vi "GUI_AndorCamera.vi"() -> ()   [LabVIEW 2020]
uses:
  Shared/GUI_Template/GUI_master/tcp_new_data_event.ctl
  Shared/GUI_Template/GUI_master/tcp new data cluster.ctl
  <vilib>/vision/NI_Vision_Development_Module.lvlib
panel:
  in  "multiplier":dbl=1.0 format="%.2f"
  in  "Refresh Button":bool
  in  "Select device":string(combo)="PL1-PresCtl"
  out "Waveform Chart":sgl(graph)
  in  "trigger::1":enum16{"Internal", "External"}(ring) caption="trigger"
  in  "pulsewidth::1":dbl caption="Pulse Width (ns)" min=0.0 max=1000000000.0
  in  "gain::1":dbl caption="gain" min=0.0 max=4095.0
  in  "temperature::1":dbl caption="Temperature (C)" min=-40.0 max=20.0
  in  "acqready::1":enum16{"yes", "no"}(ring)
  in  "stop":bool
  in  "GUIdevice 1":string="P2-AndorCam"
  out "tcp data event":T1
  in  "Tab Control":enum32{"original", "Scaled", "As Graph"}(tab)
  out "image::1":T2(plugin-control) caption="Andor Camera"
  out "andorscaled":T2(plugin-control) caption="Andor Camera"
  out "Intensity Graph":u8[][](graph)
  # "To get chart to plot, select an roi on scaled image"
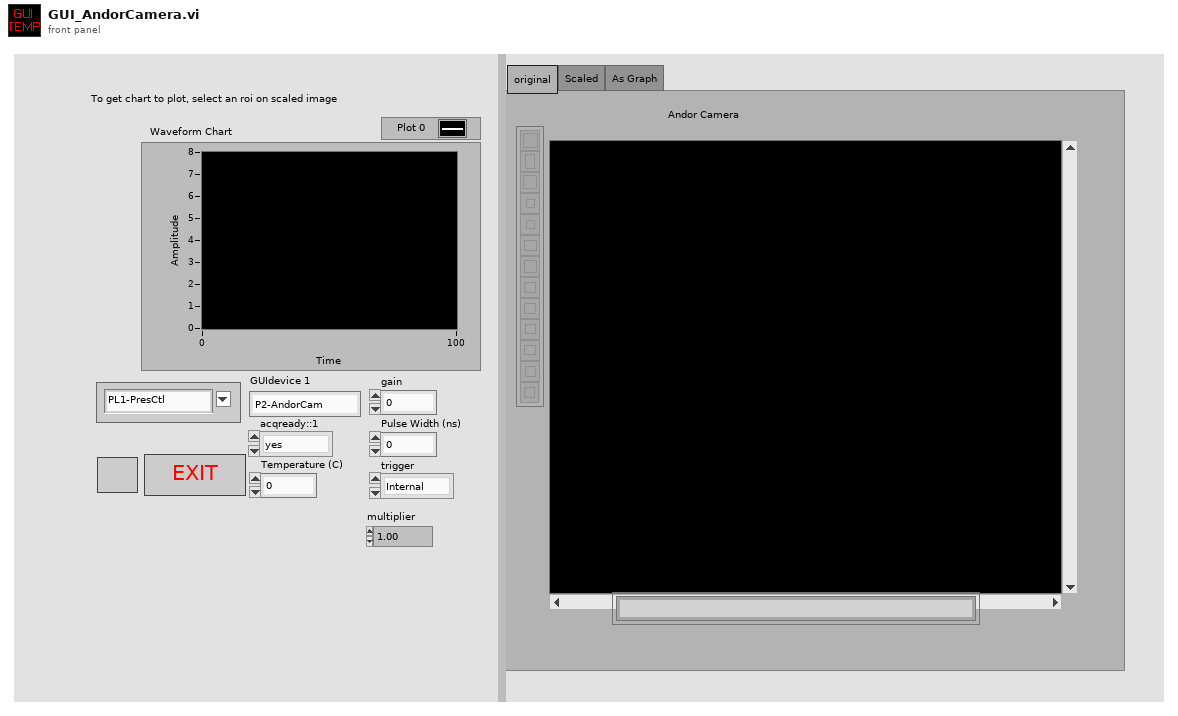
[diagram p1: front panel]
types:
  T1 = typedef "tcp_new_data_event.ctl" = refnum<user-event>
  T2 = typedef "IMAQ Image.ctl" = refnum<image>
  T3 = typedef "Image Type" = u32
  T4 = enum32{"invalid app kind", "Development System", "Run Time System", "Student Edition", "Embedded LabVIEW", "Evaluation", "Custom"}
  T5 = typedef "tcp new data cluster.ctl" = cluster{"EventEnum":enum16{"new data", "connection status update"}, "Device name":string}
  T6 = enum32{"Invalid", "Standard", "Closed", "Hidden", "Minimized", "Maximized"}
  T7 = cluster{"Core":cluster{"Current VI Reference":refnum<vi>, "Close Panel on Exit?":bool}, "SuperGUI":cluster{"STOP queue":refnum<queue>, "SuperGUI ref":refnum<vi>}}
  T8 = cluster{"STOP queue":refnum<queue>, "SuperGUI ref":refnum<vi>}
  T9 = cluster{"Current VI Reference":refnum<vi>, "Close Panel on Exit?":bool}
  T10 = cluster{"Global Rectangle":i32[], "Contours":cluster{"Contour Type":u32, "ROI Type":u32, "Points":i32[]}[]}
  T11 = cluster{"histogram":u32[], "Minimal Value":sgl, "Maximal Value":sgl, "Starting Value":sgl, "Interval Width":sgl, "Mean Value":sgl, "Standard  Variation":sgl, "Area (pixels)":i32}
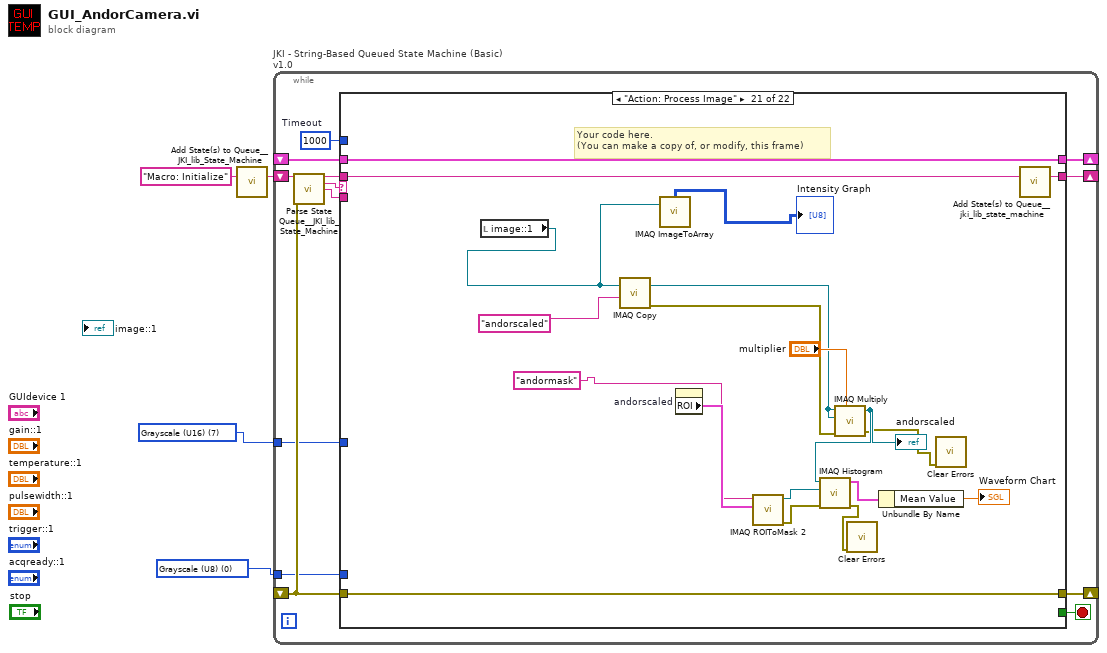
[diagram p0: block diagram]
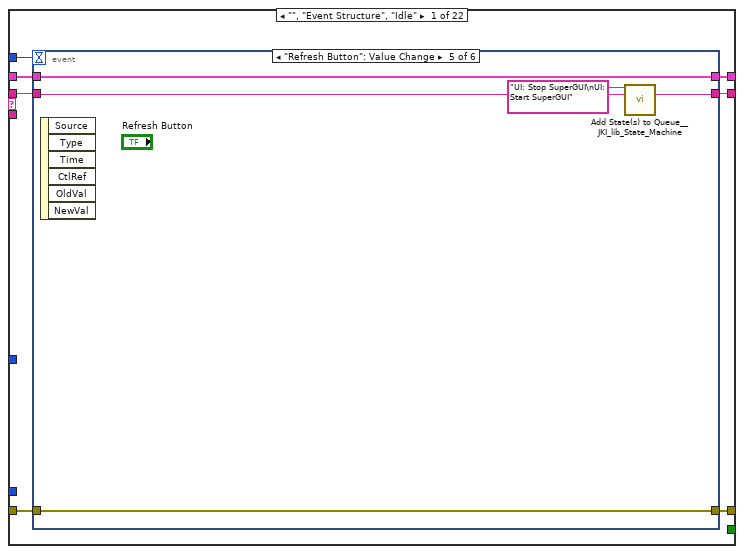
[diagram p2: hidden frame]
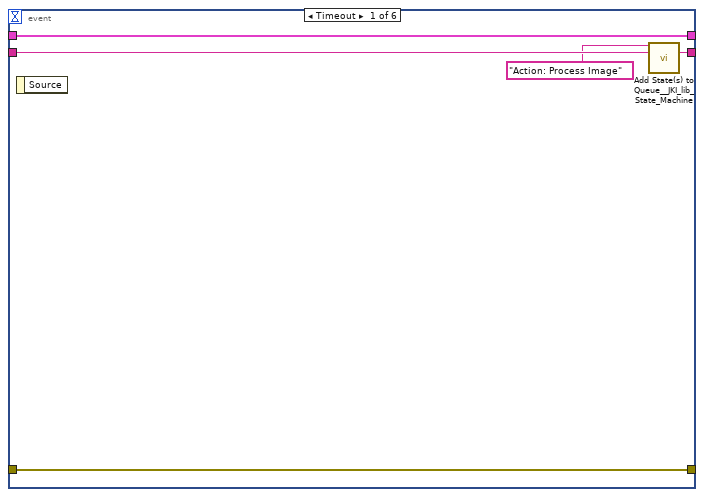
[diagram p3: hidden frame]
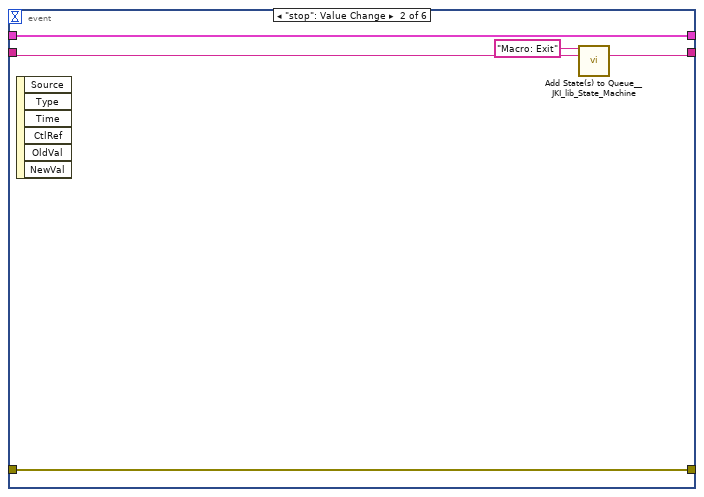
[diagram p4: hidden frame]
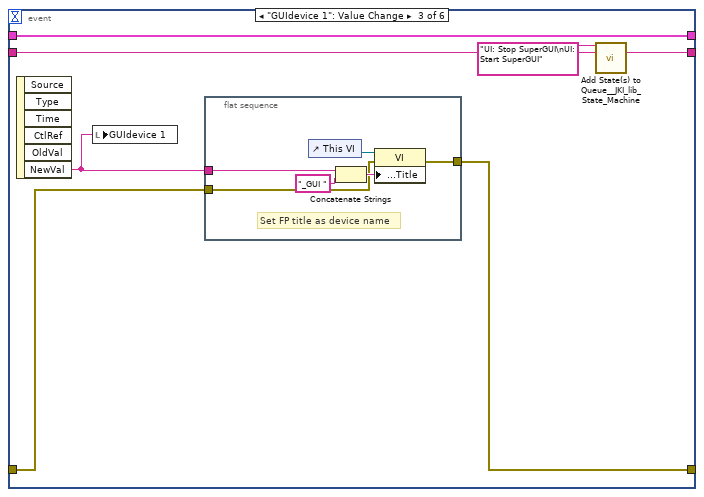
[diagram p5: hidden frame]
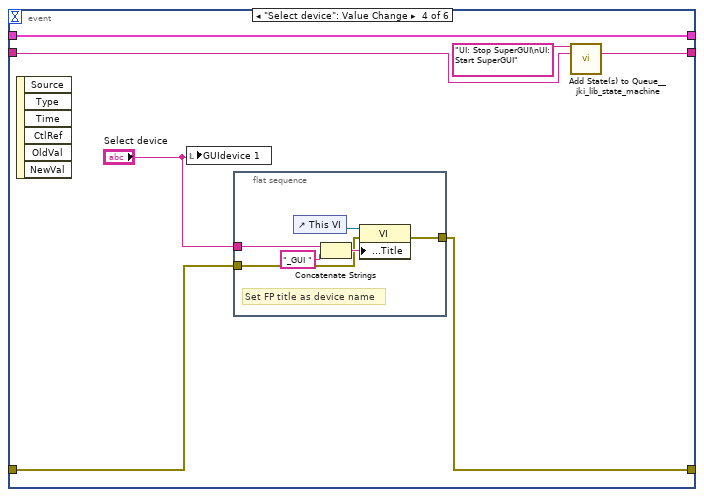
[diagram p6: hidden frame]
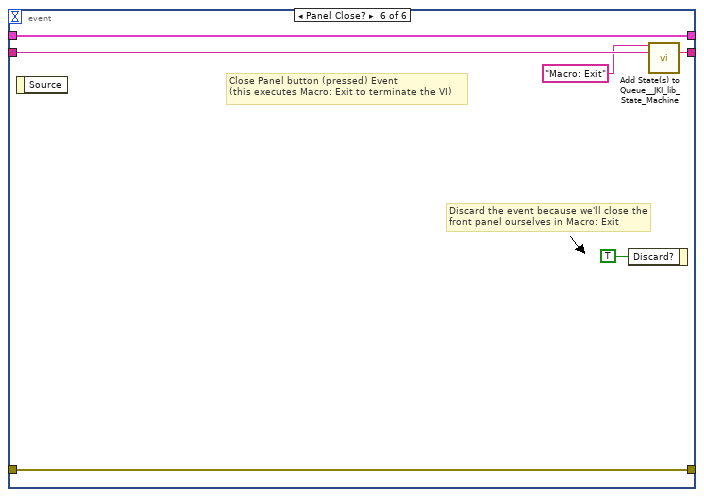
[diagram p7: hidden frame]
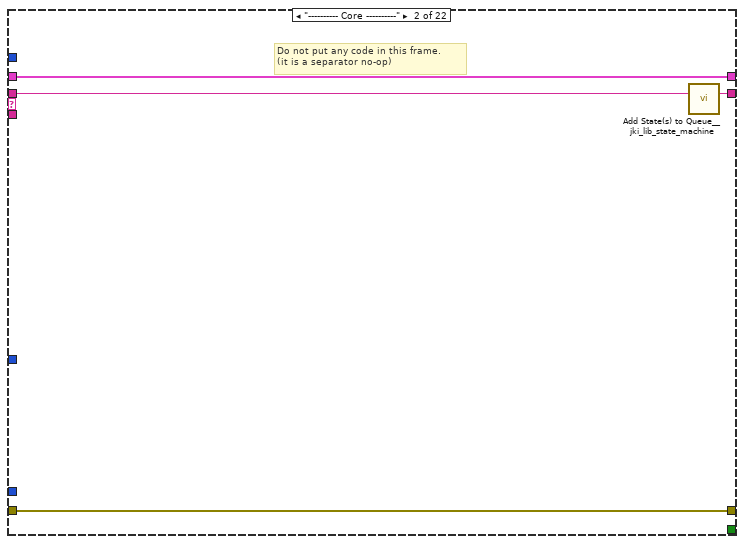
[diagram p8: hidden frame]
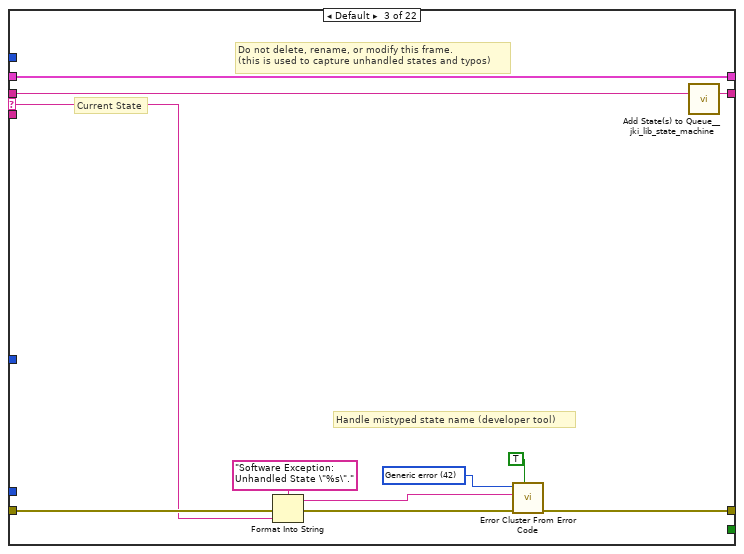
[diagram p9: hidden frame]
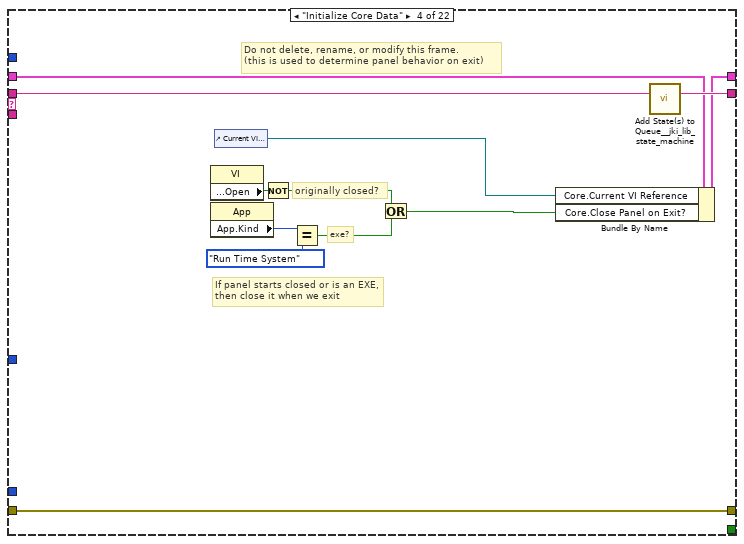
[diagram p10: hidden frame]
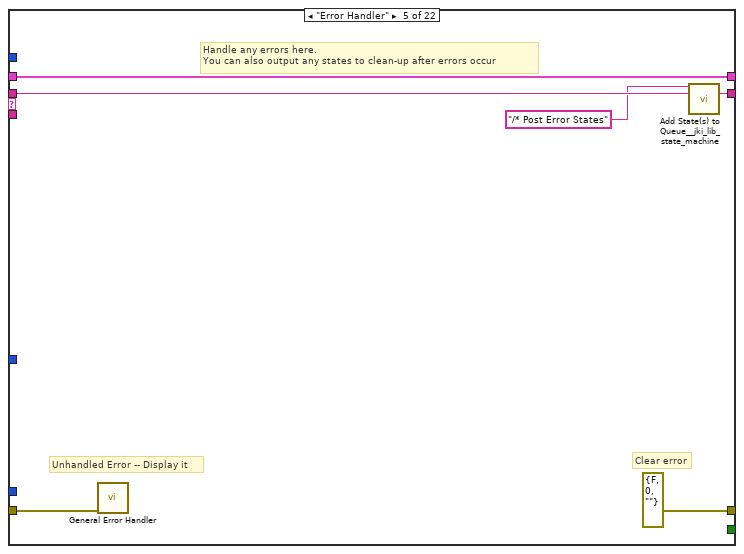
[diagram p11: hidden frame]
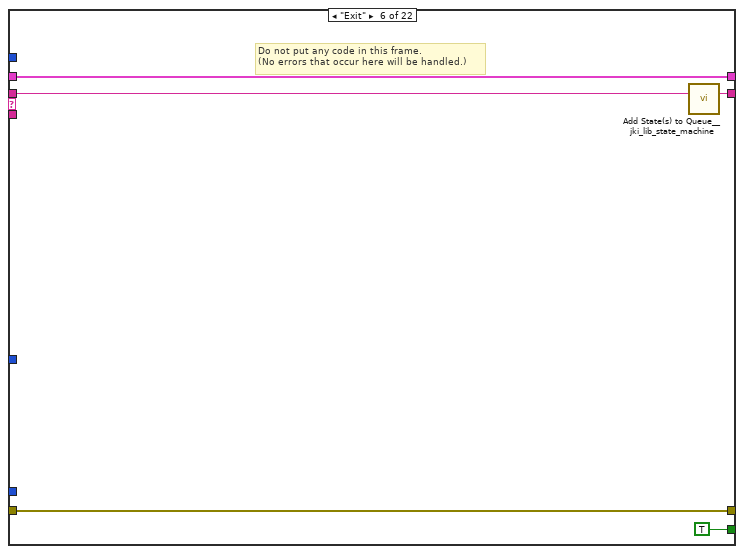
[diagram p12: hidden frame]
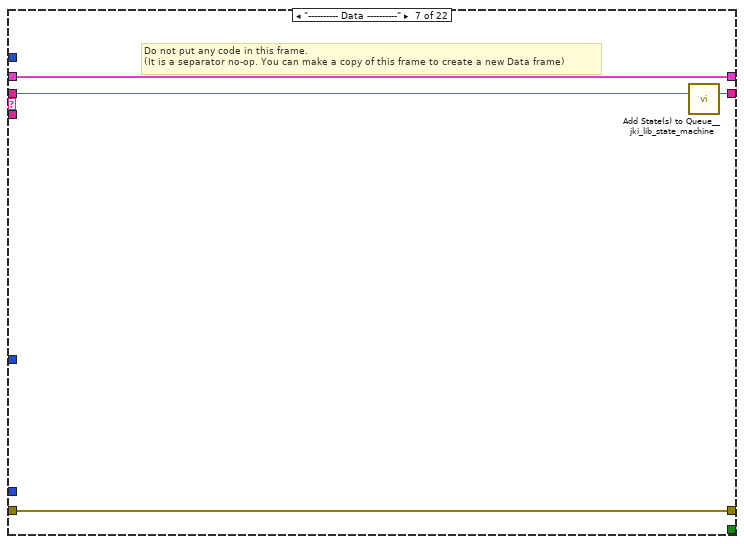
[diagram p13: hidden frame]
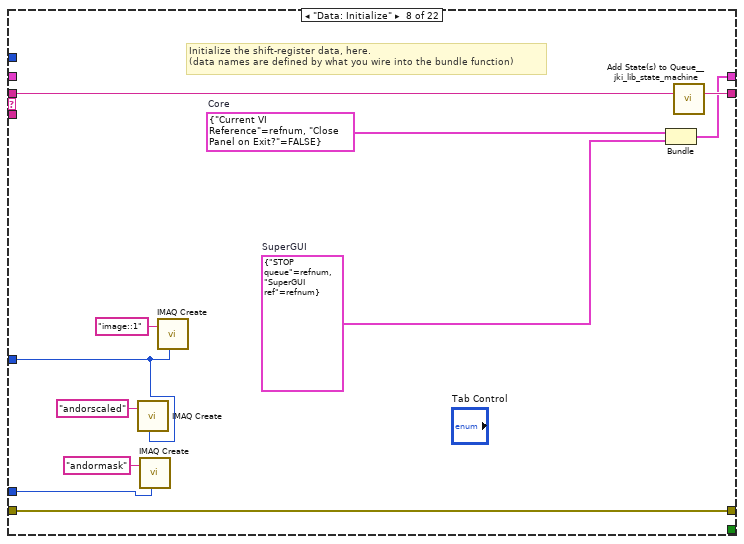
[diagram p14: hidden frame]
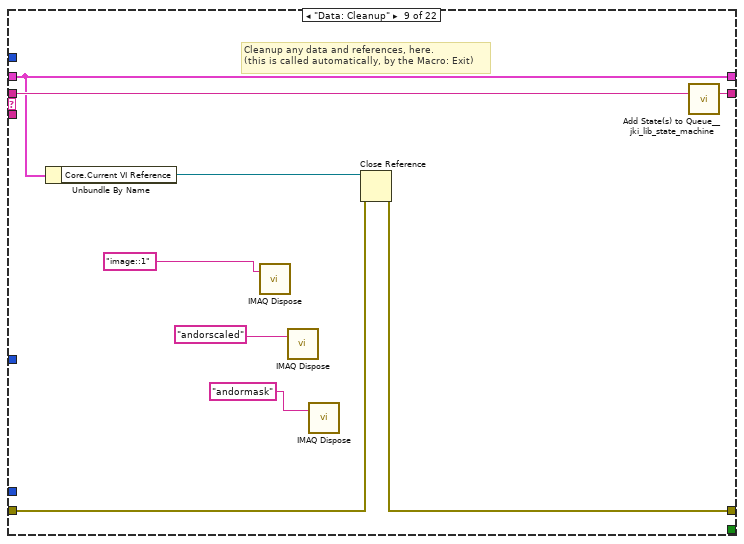
[diagram p15: hidden frame]
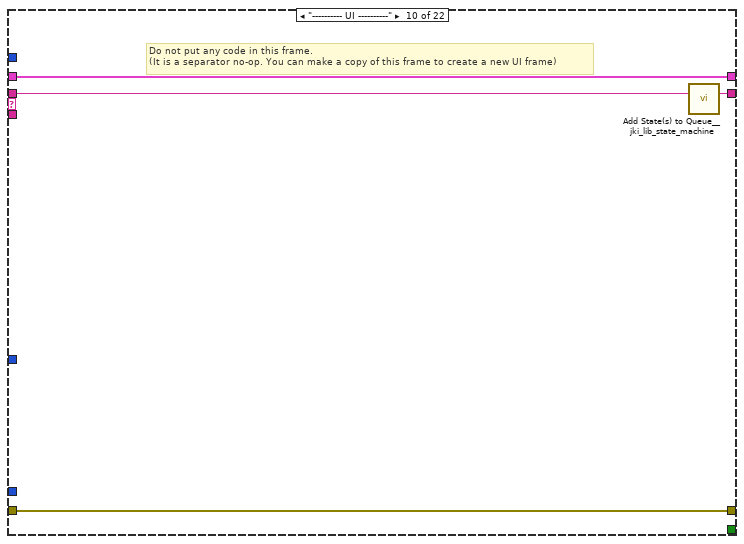
[diagram p16: hidden frame]
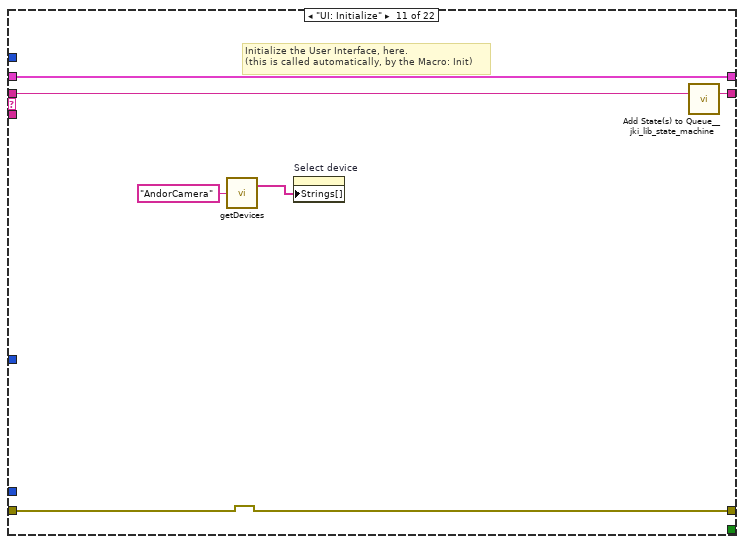
[diagram p17: hidden frame]
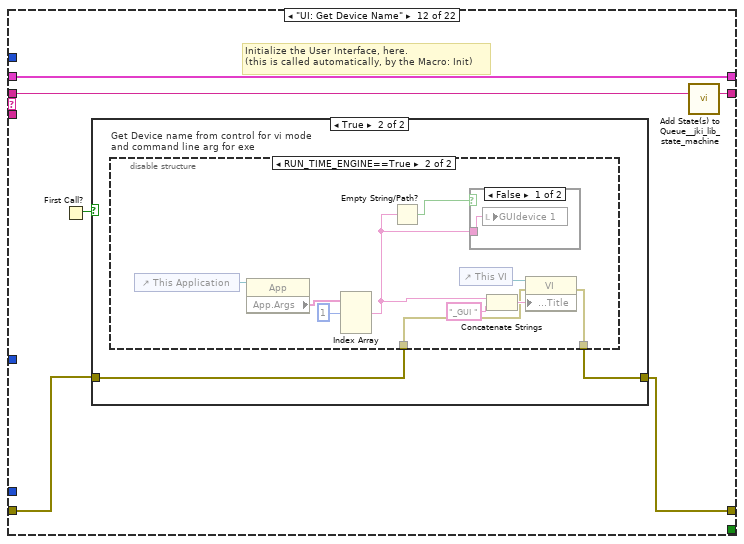
[diagram p18: hidden frame]
diagram:
  w1 = T3 0 items=["Grayscale (U8)", "Grayscale (I16)", "Grayscale (SGL)", "Complex (CSG)", "RGB (U32)", "HSL (U32)", "RGB (U64)", "Grayscale (U16)"] ("Image Type")
  w2 = T3 7 items=["Grayscale (U8)", "Grayscale (I16)", "Grayscale (SGL)", "Complex (CSG)", "RGB (U32)", "HSL (U32)", "RGB (U64)", "Grayscale (U16)"] ("Image Type")
  n1 = call <vilib>:"Add State(s) to Queue__JKI_lib_State_Machine.vi"("State(s) in (\"\")"="Macro: Initialize") -> ("States Out"=w4:string)  [unwired: 14 in]
  n2 = while "JKI - String-Based Queued State Machine (Basic) v1.0" {
    shift-right: [w10] -> _
    shift-left: _ -> [w9]
    shift-right: [w13] -> _
    shift-left: _ -> [w7]
    shift-right: [w12] -> _
    shift-left: w4 -> [w14]
    tunnel: w2 -> [w6]
    tunnel: w1 -> [w5]
    stop <- w11 stop-if-true
    w8 = 1000  # Timeout
    n3 = call <vilib>:"Parse State Queue__JKI_lib_State_Machine.vi"("State Queue"=w14, "Error In (no error)"=w7) -> ("Remaining States"=w16:string, "Current State"=w17:string, "Arguments"=w15:string)  [unwired: 11 in]
    n4 = case shown="\"Action: Process Image\"" w17 {
      selector: w17 -> [_ _ w76 _ _ _ _ _ _ _ _ _ _ _ _ _ _ _ _ _ _ _]
      tunnel: w16 -> [w24 w75 w80 w98 w104 w109 w113 w124 w133 w137 w143 w149 w184 w192 w198 w209 w235 w240 w250 w254 w273 w277]
      tunnel: w15 -> [_ _ _ _ _ _ _ _ _ _ _ _ _ _ w193 w203 _ _ _ _ _ _]
      tunnel: w9 -> [w22 w72 w78 w89 w101 w107 w110 _ w128 w134 w141 w147 w175 w187 w196 w205 w232 w237 w247 w251 w270 w274]
      tunnel: [w21 w73 w82 w95 errorcluster {"status"=FALSE, "code"=0, "source"=""} ("error out") w106 w111 w121 w129 w135 w138 w144 w168 w185 w194 w206 w233 w238 w248 w252 w271 w275] -> w13
      tunnel: w7 -> [w20 w73 w81 w95 w100 w106 w111 w121 w130 w135 w138 w145 w169 w186 w195 w207 w233 w238 w248 w252 w271 w275]
      tunnel: [w23 w74 w79 w97 w103 w108 w112 w123 w132 w136 w142 w148 w183 w191 w197 w208 w234 w239 w249 w253 w272 w276] -> w12
      tunnel: [_ _ _ _ _ TRUE _ _ _ _ _ _ _ _ _ _ _ _ _ _ _ _] -> w11
      tunnel: [w19 w72 w78 w96 w101 w107 w110 w122 w128 w134 w141 w147 w174 w187 w196 w205 w232 w237 w247 w251 w270 w274] -> w10
      tunnel: w8 -> [w18 _ _ _ _ _ _ _ _ _ _ _ _ _ _ _ _ _ _ _ _ _]
      tunnel: w6 -> [_ _ _ _ _ _ _ w115 _ _ _ _ _ _ _ _ _ _ _ _ _ _]
      tunnel: w5 -> [_ _ _ _ _ _ _ w114 _ _ _ _ _ _ _ _ _ _ _ _ _ _]
      frame "", "Event Structure", "Idle" {
        n5 = event shown="[4] \"Refresh Button\": Value Change" {
          selector: _ -> [_ _ _ _ _ _]
          dyn-events: _ -> [_ _ _ _ _ _]
          timeout: w18 -> [_ _ _ _ _ _]
          tunnel: w24 -> [w29 w32 w38 w49 w63 w71]
          tunnel: [w28 w31 w37 w48 w62 w70] -> w23
          tunnel: w22 -> [w26 w34 w41 w54 w65 w68]
          tunnel: [w27 w33 w39 w51 w64 w69] -> w21
          tunnel: w20 -> [w27 w33 w40 w52 w64 w69]
          tunnel: [w26 w34 w41 w54 w65 w68] -> w19
          event Timeout {
            n6 = event-data() -> ()  [unwired: 1 in, 1 out]
            n7 = call <vilib>:"Add State(s) to Queue__JKI_lib_State_Machine.vi"("State(s) in Front (\"\")"="Action: Process Image" ("State(s) in Front (\"\")"), "State(s) in (\"\")"=w29) -> ("States Out"=w28:string)  [unwired: 13 in]
          }
          event "stop": Value Change {
            n8 = event-data() -> ()  [unwired: 1 in, 6 out]
            n9 = call <vilib>:"Add State(s) to Queue__JKI_lib_State_Machine.vi"("State(s) in Front (\"\")"="Macro: Exit", "State(s) in (\"\")"=w32) -> ("States Out"=w31:string)  [unwired: 13 in]
          }
          event "GUIdevice 1": Value Change {
            n10 = event-data() -> ("NewVal"=w35:string)  [unwired: 1 in, 5 out]
            n11 = local write "GUIdevice 1"(w35) -> ()
            n12 = flat-sequence {
              tunnel: [w44] -> w39
              tunnel: w40 -> [w43]
              tunnel: w35 -> [w42]
              frame #0 {
                # "Set FP title as device name"
                n13 = control-ref of="This VI"() -> (w47:refnum<vi>)
                n14 = Concatenate Strings(w42, "_GUI ") -> (w46:string)
                n15 = property class="VI"(reference=w47, error in=w43, "Front Panel.Title"=w46) -> (error out=w44:errorcluster)  [unwired: 1 out]
              }
            }
            n16 = call <vilib>:"Add State(s) to Queue__JKI_lib_State_Machine.vi"("State(s) in Front (\"\")"="UI: Stop SuperGUI\nUI: Start SuperGUI", "State(s) in (\"\")"=w38) -> ("States Out"=w37:string)  [unwired: 13 in]
          }
          event "Select device": Value Change {
            n17 = event-data() -> ()  [unwired: 1 in, 6 out]
            n18 = local write "GUIdevice 1"("Select device") -> ()
            n19 = flat-sequence {
              tunnel: [w57] -> w51
              tunnel: w52 -> [w56]
              tunnel: "Select device" -> [w55]
              frame #0 {
                # "Set FP title as device name"
                n20 = control-ref of="This VI"() -> (w60:refnum<vi>)
                n21 = Concatenate Strings(w55, "_GUI ") -> (w59:string)
                n22 = property class="VI"(reference=w60, error in=w56, "Front Panel.Title"=w59) -> (error out=w57:errorcluster)  [unwired: 1 out]
              }
            }
            n23 = call <vilib>:"Add State(s) to Queue__jki_lib_state_machine.vi"("State(s) in Front (\"\")"="UI: Stop SuperGUI\nUI: Start SuperGUI", "State(s) in (\"\")"=w49) -> ("States Out"=w48:string)  [unwired: 13 in]
          }
          event "Refresh Button": Value Change {
            n24 = event-data() -> ()  [unwired: 1 in, 6 out]
            n25 = call <vilib>:"Add State(s) to Queue__JKI_lib_State_Machine.vi"("State(s) in Front (\"\")"="UI: Stop SuperGUI\nUI: Start SuperGUI", "State(s) in (\"\")"=w63) -> ("States Out"=w62:string)  [unwired: 13 in]
          }
          event Panel Close? {
            # "Discard the event because we'll close the front panel ourselves in Macro: Exit"
            # "Close Panel button (pressed) Event\n(this executes Macro: Exit to terminate the VI)"
            n26 = event-data() -> ()  [unwired: 1 in, 1 out]
            n27 = event-data("Discard?"=TRUE) -> ()  [unwired: 1 in, 1 out]
            n28 = call <vilib>:"Add State(s) to Queue__JKI_lib_State_Machine.vi"("State(s) in Front (\"\")"="Macro: Exit", "State(s) in (\"\")"=w71) -> ("States Out"=w70:string)  [unwired: 13 in]
          }
        }
      }
      frame "---------- Core ----------" {
        # "Do not put any code in this frame.\n(it is a separator no-op)"
        n29 = call <vilib>:"Add State(s) to Queue__jki_lib_state_machine.vi"("State(s) in (\"\")"=w75) -> ("States Out"=w74:string)  [unwired: 14 in]
      }
      frame Default {
        w85 = 42 items=["No error", "Argument error", "Memory is full", "Out of zone", "End of file", "File already open", "Generic file I/O error", "File not found", "File permission error", "Disk is full", "Duplicate path", "Too many files open", "System feature not enabled", "Resource file not found", "Cannot add resource", "Resource not found", "Image not found", "Image memory error", "Pen does not exist", "Config type invalid", "Config token not found", "Config parse error", "Config memory error", "Bad external code format", "Bad external code offset", "External code not present", "Null window", "Destroy window error", "Null menu", "Print aborted", "Bad print record", "Print driver error", "Windows error during printing", "Memory error during printing", "Print dialog error", "Generic print error", "Invalid device refnum", "Device not found", "Device parameter error", "Device unit error", "Cannot open device", "Device call aborted", "Generic error", "Cancelled by user", "Object ID too low", "Object ID too high", "Object not in heap", "Unknown heap", "Unknown object (invalid DefProc)", "Unknown object (DefProc not in table)", "Message out of range", "Invalid (null) method", "Unknown message", "Manager call not supported", "Bad address", "Network operation in progress", "Network operation timed out", "Connection is busy", "Network attribute not supported", "Network error", "Address in use", "System out of memory", "Connection aborted", "Connection refused", "Not connected", "Already connected", "Connection closed", "Initialization error (interapplication manager)", "Bad occurrence", "Wait on unbound occurrence handler", "Occurrence queue overflow", "Datalog type conflict", "Unused", "Unrecognized type (interapplication manager)", "Memory corrupt", "Failed to make temporary DLL", "Old CIN version", "Drag socket not found", "Failed to load drop-object", "Failed to register OLE object", "Failed to release OLE object", "Format specifier type mismatch", "Unknown format specifier", "Too few format specifiers", "Too many format specifiers", "Scan failed", "Newer CIN version", "Error converting to variant", "Runtime menu error", "Password tampered", "Variant attribute not found", "Incompatible variant data type", "Event data is not available", "Event Store is not present", "Occurrence is not found", "Event Queue is not created", "Event info is not available", "Refnum passed is NULL", "Error retrieving Class GUID", "Error retrieving CoClass GUID", "Error retrieving TypeLib GUID.", "Bad built application magic bytes.", "Specific driver is different from the specific driver associated with the Logical Name.", "There is no session opened to the class driver.", "Max Error", "MAX - Error with config objects", "MAX - Error loading configuration", "MAX - Group not supported"]
        # "Current State"
        # "Do not delete, rename, or modify this frame.\n(this is used to capture unhandled states and typos)"
        # "Handle mistyped state name (developer tool)"
        n30 = Format Into String(format string="Software Exception: Unhandled State \"%s\"." ("message"), error in=w81, w76) -> (resulting string=w84:string, error out=w83:errorcluster)  [unwired: 1 in]
        n31 = call <vilib>:"Error Cluster From Error Code.vi"("show call chain? (False)"=TRUE, "error in (no error)"=w83, "error message (\"\")"=w84, "error code (0)"=w85) -> ("error out"=w82:errorcluster)  [unwired: 5 in]
        n32 = call <vilib>:"Add State(s) to Queue__jki_lib_state_machine.vi"("State(s) in (\"\")"=w80) -> ("States Out"=w79:string)  [unwired: 14 in]
      }
      frame "Initialize Core Data" {
        # "Do not delete, rename, or modify this frame.\n(this is used to determine panel behavior on exit)"
        # "originally closed?"
        # "exe?"
        # "If panel starts closed or is an EXE, then close it when we exit"
        n33 = property class="VI"() -> ("Front Panel.Open"=w94:bool)  [unwired: 2 in, 2 out]
        n34 = property class="App"() -> ("App.Kind"=w93:T4)  [unwired: 2 in, 2 out]
        n35 = control-ref of="Current VI Reference"() -> (w87:refnum<vi>)
        n36 = Not(x=w94) -> (.not. x?=w91:bool)
        n37 = Equal?(x=w93, y=T4."Run Time System" ("Application:Kind")) -> (x = y?=w90:bool)
        n38 = Or(x=w91, y=w90) -> (x .or. y?=w88:bool)
        n39 = Bundle By Name(cluster=w89, "Core.Current VI Reference"=w87, "Core.Close Panel on Exit?"=w88) -> (w96:T7)
        n40 = call <vilib>:"Add State(s) to Queue__jki_lib_state_machine.vi"("State(s) in (\"\")"=w98) -> ("States Out"=w97:string)  [unwired: 14 in]
      }
      frame "Error Handler" {
        # "Unhandled Error -- Display it"
        # "Handle any errors here.\nYou can also output any states to clean-up after errors occur"
        # "Clear error"
        n41 = call <vilib>:"General Error Handler.vi"("error in (no error)"=w100) -> ()  [unwired: 10 in, 5 out]
        n42 = call <vilib>:"Add State(s) to Queue__jki_lib_state_machine.vi"("State(s) in Front (\"\")"="/* Post Error States", "State(s) in (\"\")"=w104) -> ("States Out"=w103:string)  [unwired: 13 in]
      }
      frame "Exit" {
        # "Do not put any code in this frame.\n(No errors that occur here will be handled.)"
        n43 = call <vilib>:"Add State(s) to Queue__jki_lib_state_machine.vi"("State(s) in (\"\")"=w109) -> ("States Out"=w108:string)  [unwired: 14 in]
      }
      frame "---------- Data ----------" {
        # "Do not put any code in this frame.\n(It is a separator no-op. You can make a copy of this frame to create a new Data frame)"
        n44 = call <vilib>:"Add State(s) to Queue__jki_lib_state_machine.vi"("State(s) in (\"\")"=w113) -> ("States Out"=w112:string)  [unwired: 14 in]
      }
      frame "Data: Initialize" {
        w119 = T8 {"STOP queue"=refnum, "SuperGUI ref"=refnum}  # SuperGUI
        w120 = T9 {"Current VI Reference"=refnum, "Close Panel on Exit?"=FALSE}  # Core
        # "Initialize the shift-register data, here.\n(data names are defined by what you wire into the bundle function)"
        n45 = call "IMAQ Create"("Image Name"="andorscaled", "Image Type"=w115) -> ()  [unwired: 3 in, 2 out]
        n46 = call "IMAQ Create"("Image Name"="andormask", "Image Type"=w114) -> ()  [unwired: 3 in, 2 out]
        n47 = call "IMAQ Create"("Image Name"="image::1", "Image Type"=w115) -> ()  [unwired: 3 in, 2 out]
        n48 = Bundle("Core"=w120, "SuperGUI"=w119) -> (w122:T7)  [unwired: 1 in]
        n49 = call <vilib>:"Add State(s) to Queue__jki_lib_state_machine.vi"("State(s) in (\"\")"=w124) -> ("States Out"=w123:string)  [unwired: 14 in]
      }
      frame "Data: Cleanup" {
        # "Cleanup any data and references, here.\n(this is called automatically, by the Macro: Exit)"
        n50 = Unbundle By Name(w128) -> ("Core.Current VI Reference"=w131:refnum<vi>)
        n51 = call "IMAQ Dispose"("Image"="image::1" ("Image Name")) -> ()  [unwired: 5 in, 1 out]
        n52 = call "IMAQ Dispose"("Image"="andorscaled" ("Image Name")) -> ()  [unwired: 5 in, 1 out]
        n53 = call "IMAQ Dispose"("Image"="andormask" ("Image Name")) -> ()  [unwired: 5 in, 1 out]
        n54 = Close Reference(reference=w131, error in (no error)=w130) -> (error out=w129:errorcluster)
        n55 = call <vilib>:"Add State(s) to Queue__jki_lib_state_machine.vi"("State(s) in (\"\")"=w133) -> ("States Out"=w132:string)  [unwired: 14 in]
      }
      frame "---------- UI ----------" {
        # "Do not put any code in this frame.\n(It is a separator no-op. You can make a copy of this frame to create a new UI frame)"
        n56 = call <vilib>:"Add State(s) to Queue__jki_lib_state_machine.vi"("State(s) in (\"\")"=w137) -> ("States Out"=w136:string)  [unwired: 14 in]
      }
      frame "UI: Initialize" {
        # "Initialize the User Interface, here.\n(this is called automatically, by the Macro: Init)"
        n57 = call "getDevices.vi"("Device Class"="AndorCamera") -> ("All Devices"=w139:string[])  [unwired: 1 out]
        n58 = property on="Select device" class="CmbBox"("Strings[]"=w139) -> ()  [unwired: 2 in, 2 out]
        n59 = call <vilib>:"Add State(s) to Queue__jki_lib_state_machine.vi"("State(s) in (\"\")"=w143) -> ("States Out"=w142:string)  [unwired: 14 in]
      }
      frame "UI: Get Device Name" {
        # "Initialize the User Interface, here.\n(this is called automatically, by the Macro: Init)"
        n60 = First Call?() -> (First Call?: T/F=w146:bool)
        n61 = case shown="True" w146 {
          tunnel: w145 -> [w150 w152]
          tunnel: [w150 w151] -> w144
          frame False {
          }
          frame True {
            n62 = disable-structure "Get Device name from control for vi mode\nand command line arg for exe" shown="RUN_TIME_ENGINE==True" {
              disable-tunnel: w152 -> [w153 w155]
              disable-tunnel: [w153 w154] -> w151
              frame condition #0 (active) {
              }
              frame condition #1 {
                n63 = control-ref of="This Application"() -> (w163:refnum<vi>)
                n64 = property class="App"(reference=w163) -> ("App.Args"=w162:string[])  [unwired: 1 in, 2 out]
                n65 = Index Array(array=w162, index #1=1 ("index")) -> (element #1=w156:string)  [unwired: 2 in, 2 out]
                n66 = Empty String/Path?(string/path=w156) -> (empty?=w160:bool)
                n67 = control-ref of="This VI"() -> (w159:refnum<vi>)
                n68 = case shown="False" w160 {
                  tunnel: w156 -> [w164 _]
                  frame False {
                    n69 = local write "GUIdevice 1"(w164) -> ()
                  }
                  frame True {
                  }
                }
                n70 = Concatenate Strings(w156, "_GUI ") -> (w158:string)
                n71 = property class="VI"(reference=w159, error in=w155, "Front Panel.Title"=w158) -> (error out=w154:errorcluster)  [unwired: 1 out]
              }
            }
          }
        }
        n72 = call <vilib>:"Add State(s) to Queue__jki_lib_state_machine.vi"("State(s) in (\"\")"=w149) -> ("States Out"=w148:string)  [unwired: 14 in]
      }
      frame "UI: Start SuperGUI" {
        # "create stop queue for supergui and its clones"
        # "x100 abort will be dependent on caller VI\nx80 abort will be independent of caller vi, this will abort vi when labview is closed."
        # "Start SuperGUI asynchronous way"
        n73 = vi-ref "GUI_Master_subvi_reentrant_queues.vi"() -> (w167:refnum<vi>)
        n74 = property class="VI"(reference=w167) -> ("Path"=w166:path)  [unwired: 1 in, 2 out]
        n75 = Create User Event(user event datatype=T5 {"EventEnum"=enum."new data", "Device name"="Device name"} ("New Event"), error in=w169) -> (user event=w170:refnum<user-event>, error out=w176:errorcluster)
        "tcp data event" <- w170
        n76 = control-ref of="This Application"() -> (w173:refnum<vi>)
        n77 = control-ref of="This VI"() -> (w172:refnum<vi>)
        n78 = Open VI Reference(type specifier VI Refnum (for type only)=refnum<vi> refnum, vi path=w166, options=256) -> (vi reference=w182:refnum<vi>, error out=w181:errorcluster)  [unwired: 3 in]
        n79 = register-events(w170) -> ()  [unwired: 2 in, 2 out]
        n80 = call "supergui create stop queue.vi"() -> ("STOP Queue out"=w178:refnum<queue>)  [unwired: 11 in]
        n81 = Current VI's Menubar() -> (w171:refnum<k9>)
        n82 = call-by-ref "Start Asynchronous Call"(reference=w182, error in=w181, "STOP Queue in"=w178, "This Application"=w173, 8:"error in (no error)"=w176, "tcp data event"=w170, "Caller menu reference"=w171, "Caller VI ref"=w172) -> (reference out=w165:refnum<vi>, error out=w168:errorcluster)  [unwired: 5 in, 1 out]
        n83 = Bundle By Name(cluster=w175, "SuperGUI.SuperGUI ref"=w165, "SuperGUI.STOP queue"=w178) -> (w174:T7)
        n84 = call <vilib>:"Add State(s) to Queue__jki_lib_state_machine.vi"("State(s) in (\"\")"=w184) -> ("States Out"=w183:string)  [unwired: 14 in]
      }
      frame "UI: Stop SuperGUI" {
        # "Stop Supergui Clone and wait until it exit properly"
        n85 = Unbundle By Name(w187) -> ("SuperGUI.SuperGUI ref"=w189:refnum<vi>, "SuperGUI.STOP queue"=w188:refnum<queue>)
        n86 = Release Queue(queue=w188, error in (no error)=w186) -> (error out=w190:errorcluster)  [unwired: 1 in, 2 out]
        n87 = call-by-ref "Wait On Asynchronous Call"(reference=w189, error in=w190) -> ("error out"=w185:errorcluster)  [unwired: 11 in, 2 out]
        n88 = call <vilib>:"Add State(s) to Queue__jki_lib_state_machine.vi"("State(s) in (\"\")"=w192) -> ("States Out"=w191:string)  [unwired: 14 in]
      }
      frame "UI: Cursor Set" {
        # "Argument"
        # "Set and Unset Cursor Busy.\n(Usage: \"UI: Cursor Set >> Busy|Idle\")"
        n89 = case shown="\"Idle\", Default" w193 {
          tunnel: w195 -> [w200 w202]
          tunnel: [w199 w201] -> w194
          frame "Idle", Default {
            n90 = call <vilib>:"Unset Busy.vi"("error in (no error)"=w200) -> ("error out"=w199:errorcluster)  [unwired: 10 in]
          }
          frame "Busy" {
            n91 = call <vilib>:"Set Busy.vi"("error in (no error)"=w202) -> ("error out"=w201:errorcluster)  [unwired: 9 in, 1 out]
          }
        }
        n92 = call <vilib>:"Add State(s) to Queue__jki_lib_state_machine.vi"("State(s) in (\"\")"=w198) -> ("States Out"=w197:string)  [unwired: 14 in]
      }
      frame "UI: Front Panel State" {
        # "Argument"
        # "Set Front Panel Open or Closed\n(Usage: \"UI: Front Panel State >> Open|Close\")"
        n93 = Unbundle By Name(w205) -> ("Core.Current VI Reference"=w204:refnum<vi>)
        n94 = case shown="\"Open\", Default" w203 {
          tunnel: w207 -> [w213 w226]
          tunnel: [w215 w227] -> w206
          tunnel: w204 -> [w214 w224]
          frame "Open", Default {
            n95 = property class="VI"(reference=w214, error in=w213) -> (reference out=w211:refnum<vi>, error out=w212:errorcluster, "Front Panel.Open"=w210:bool)
            n96 = case shown="False" w210 {
              tunnel: [w218 w221] -> w215
              tunnel: w212 -> [w217 w221]
              tunnel: w211 -> [w216 _]
              frame False {
                n97 = invoke class="VI" method="FP.Open"(reference=w216, error in=w217, "Activate"=TRUE, "State"=T6."Standard") -> (error out=w218:errorcluster)  [unwired: 1 in, 4 out]
              }
              frame True {
              }
            }
          }
          frame "Close" {
            n98 = property class="VI"(reference=w224, error in=w226) -> (reference out=w223:refnum<vi>, error out=w225:errorcluster, "Front Panel.Open"=w222:bool)
            n99 = case shown="True" w222 {
              tunnel: [w228 w231] -> w227
              tunnel: w225 -> [w228 w230]
              tunnel: w223 -> [_ w229]
              frame False {
              }
              frame True {
                n100 = invoke class="VI" method="FP.Close"(reference=w229, error in=w230) -> (error out=w231:errorcluster)  [unwired: 1 in, 2 out]
              }
            }
          }
        }
        n101 = call <vilib>:"Add State(s) to Queue__jki_lib_state_machine.vi"("State(s) in (\"\")"=w209) -> ("States Out"=w208:string)  [unwired: 14 in]
      }
      frame "---------- Macro ----------" {
        # "Do not put any code in this frame.\n(It is a separator no-op. You can make a copy of this frame to create a new Macro frame)"
        n102 = call <vilib>:"Add State(s) to Queue__jki_lib_state_machine.vi"("State(s) in (\"\")"=w235) -> ("States Out"=w234:string)  [unwired: 14 in]
      }
      frame "Macro: Initialize" {
        # "Initialization Macro\n(This is called once, when the VI starts)"
        n103 = call <vilib>:"Add State(s) to Queue__jki_lib_state_machine.vi"("State(s) in Front (\"\")"="Data: Initialize\nInitialize Core Data\nUI: Initialize\nUI: Get Device Name\nUI: Start SuperGUI\nUI: Front Panel State >> Open", "State(s) in (\"\")"=w240) -> ("States Out"=w239:string)  [unwired: 13 in]
      }
      frame "Macro: Exit" {
        # "Exit Macro\n(This is called once, when the VI exits)"
        n104 = Unbundle By Name(w247) -> ("Core.Close Panel on Exit?"=w246:bool)
        n105 = Select(t="UI: Front Panel State >> Close", s=w246, f="") -> (s? t:f=w243:string)
        n106 = call <vilib>:"Add State(s) to Queue__jki_lib_state_machine.vi"("State(s) in (\"\")"=w243, "State(s) at Back (\"\")"="Data: Cleanup\nExit") -> ("States Out"=w241:string)  [unwired: 13 in]
        n107 = call <vilib>:"Add State(s) to Queue__jki_lib_state_machine.vi"("State(s) in Front (\"\")"=w241, "State(s) in (\"\")"=w250) -> ("States Out"=w249:string)  [unwired: 13 in]
      }
      frame "---------- New Category ----------" {
        # "Template Separator\n(You can make a copy of, or modify, this frame)"
        n108 = call <vilib>:"Add State(s) to Queue__jki_lib_state_machine.vi"("State(s) in (\"\")"=w254) -> ("States Out"=w253:string)  [unwired: 14 in]
      }
      frame "Action: Process Image" {
        # "Your code here.\n(You can make a copy of, or modify, this frame)"
        n109 = local read "image::1"() -> (w256:T2)
        n110 = call "IMAQ Copy"("Image Dst"="andorscaled" ("Image Name"), "Image Src"=w256) -> ("error out"=w258:errorcluster, "Image Dst Out"=w261:T2)  [unwired: 4 in]
        n111 = call "IMAQ ImageToArray"("Image"=w256) -> ("Image Pixels (U8)"=→"Intensity Graph":u8[][])  [unwired: 3 in, 4 out]
        n112 = property on="andorscaled" class="ImageControl"() -> ("ROI"=w264:T10)  [unwired: 2 in, 2 out]
        n113 = call "IMAQ ROIToMask 2"("ROI Descriptor"=w264, "Image"="andormask" ("Image Name")) -> ("error out"=w269:errorcluster, "Image Out"=w265:T2)  [unwired: 7 in, 1 out]
        n114 = call "IMAQ Multiply"("Image Src A"=w261, "Constant"="multiplier", "Image Dst"=w261, "error in (no error)"=w258) -> ("Image Dst Out"=w263:T2, "error out"=w257:errorcluster)  [unwired: 3 in]
        "andorscaled" <- w263
        n115 = call "IMAQ Histogram"("error in (no error)"=w269, "Image Mask"=w265, "Image"=w263) -> ("error out"=w268:errorcluster, "Histogram Report"=w266:T11)  [unwired: 7 in]
        n116 = call <vilib>:"Clear Errors.vi"("error in (no error)"=w268) -> ()  [unwired: 5 in, 2 out]
        n117 = Unbundle By Name(w266) -> ("Mean Value"=→"Waveform Chart":sgl)
        n118 = call <vilib>:"Clear Errors.vi"("error in (no error)"=w257) -> ()  [unwired: 5 in, 2 out]
        n119 = call <vilib>:"Add State(s) to Queue__jki_lib_state_machine.vi"("State(s) in (\"\")"=w273) -> ("States Out"=w272:string)  [unwired: 14 in]
      }
      frame "New Category: 2" {
        # "Your code here.\n(You can make a copy of, or modify, this frame)"
        n120 = call <vilib>:"Add State(s) to Queue__jki_lib_state_machine.vi"("State(s) in (\"\")"=w277) -> ("States Out"=w276:string)  [unwired: 14 in]
      }
    }
  }
